vi "Get_Initial_Value_For_Thresholding-1.vi"(0 "[IN] Histogram Graph":T1 {"Incremental Value" format="%.2f"; "Starting Value" format="%.2f"}, 1 "error IN":errorcluster) -> (2 "[OUT] Index of starting \npoint for thresholding":i32, 3 "[OUT] Minimal index for \nthresholding (negative)":i32, 4 "[OUT] Maximal index \nfor thresholding":i32, 5 "error OUT":errorcluster)   [LabVIEW 2013]
doc: "Calculation of peak value in the histogram of the LoG processed image (commonly, such histogram has the bell-shape form and always possess some peak value)"
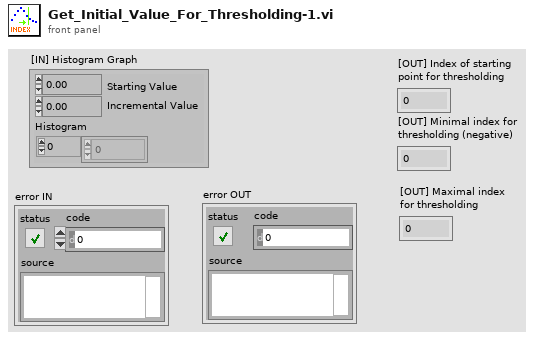
[diagram p1: front panel]
types:
  T1 = cluster{"Starting Value":sgl, "Incremental Value":sgl, "Histogram":u32[]}
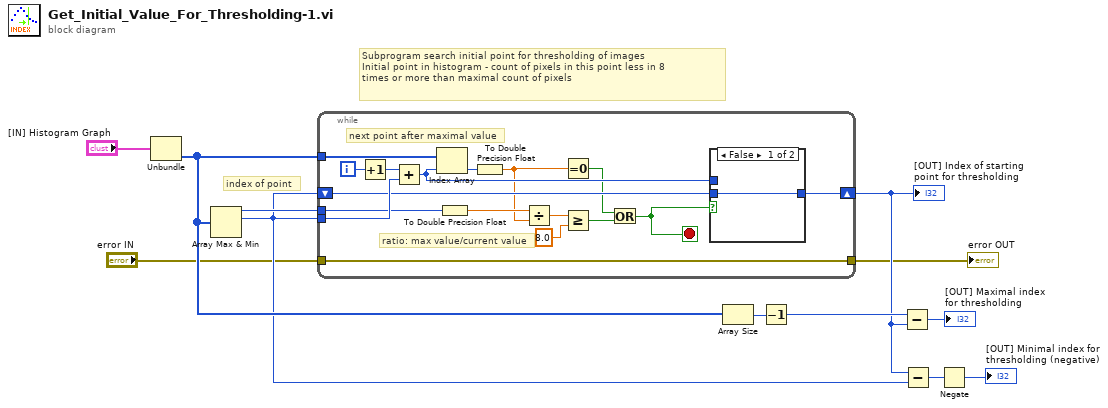
[diagram p0: block diagram]
diagram:
  # "index of point"
  # "Subprogram search initial point for thresholding of images\nInitial point in histogram - count of pixels in this point less in 8\ntimes or more than maximal count of pixels"
  n1 = Unbundle("[IN] Histogram Graph") -> ("Histogram"=w10:u32[])  [unwired: 2 out]
  n2 = Array Max & Min(array=w10) -> (max value=w11:u32, max index (indices)=w5:i32)  [unwired: 2 out]
  n3 = while {
    tunnel: w5 -> [w26]
    tunnel: w11 -> [w24]
    tunnel: w10 -> [w28]
    shift-right: [w19] -> w6
    shift-left: w5 -> [w20]
    tunnel: "error IN" -> [w13]
    tunnel: [w13] -> w1
    i -> [w29]
    stop <- w14 stop-if-true
    # "ratio: max value/current value"
    # "next point after maximal value"
    n4 = Increment(x=w29) -> (x+1=w27:i32)
    n5 = Add(x=w27, y=w26) -> (x+y=w18:i32)
    n6 = Index Array(array=w28, index=w18) -> (element=w25:u32)
    n7 = To Double Precision Float(number=w24) -> (double precision float=w23:dbl)
    n8 = To Double Precision Float(number=w25) -> (double precision float=w16:dbl)
    n9 = Divide(x=w23, y=w16) -> (x/y=w22:dbl)
    n10 = Equal To 0?(x=w16) -> (x = 0?=w15:bool)
    n11 = Greater Or Equal?(x=w22, y=8.0) -> (x >= y?=w17:bool)
    n12 = Or(x=w15, y=w17) -> (x .or. y?=w14:bool)
    n13 = case shown="False" w14 {
      tunnel: w20 -> [w30 _]
      tunnel: [w30 w31] -> w19
      tunnel: w18 -> [_ w31]
      frame False {
      }
      frame True {
      }
    }
  }
  "[OUT] Index of starting \npoint for thresholding" <- w6
  "error OUT" <- w1
  n14 = Array Size(array=w10) -> (size(s)=w9:i32)
  n15 = Decrement(x=w9) -> (x-1=w8:i32)
  n16 = Subtract(x=w8, y=w6) -> (x-y=→"[OUT] Maximal index \nfor thresholding":i32)
  n17 = Subtract(x=w6, y=w5) -> (x-y=w4:i32)
  n18 = Negate(x=w4) -> (-x=→"[OUT] Minimal index for \nthresholding (negative)":i32)
